vi "To File.vi"(8 "error in":errorcluster, 10 "Filepath":path, 11 "config-ini in":refnum<class "config-ini.lvclass">) -> (0 "error out":errorcluster, 3 "config-ini out":refnum<class "config-ini.lvclass">)   [LabVIEW 2022 SP3, in "hse-config.lvlib" / "config-ini.lvclass"]
doc: "Writes the config-ini object to an INI-file.\n\n____\nHAMPEL SOFTWARE ENGINEERING v3.8.0 (2023-12-18 14:41)"
uses:
  config-ini.lvclass
  <vilib>/Utility/config.llb/Write Key (Boolean).vi
  <vilib>/Utility/config.llb/Write Key (String).vi
  <vilib>/Utility/config.llb/Write Key (Double).vi
  <vilib>/Utility/config.llb/Write Key (I32).vi
  <vilib>/Utility/config.llb/NI_LVConfig.lvlib
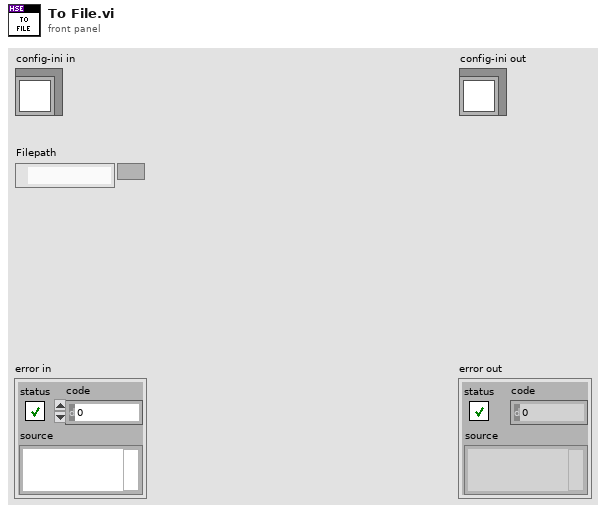
[diagram p1: front panel]
types:
  T1 = typedef "NI_LVConfig.lvlib/Config Data RefNum.ctl" = refnum<k1>
  T2 = typedef "NI_Data Type.lvlib/Data Type.ctl" = enum8{"Invalid Type", "Void", "I8", "I16", "I32", "I64", "U8", "U16", "U32", "U64", "Single Float", "Double Float", "Extended Float", "Single Complex", "Double Complex", "Extended Complex", "Enum U8", "Enum U16", "Enum U32", "Enum U64", "Single Float With Unit", "Double Float With Unit", "Extended Float With Unit", "Single Complex with Unit", "Double Complex with Unit", "Extended Complex with Unit", "Boolean", "String", "Path", "Picture", "Tag", "Array", "Cluster", "Variant", "LV Variant", "Waveform", "Timestamp", "Digital Waveform", "Digital Data", "ExpressData", "Refnum", "External Data", "VI", "Poly VI", "LabVIEW Class Instance", "Fixed Point", "Set Collection", "Map Collection"}
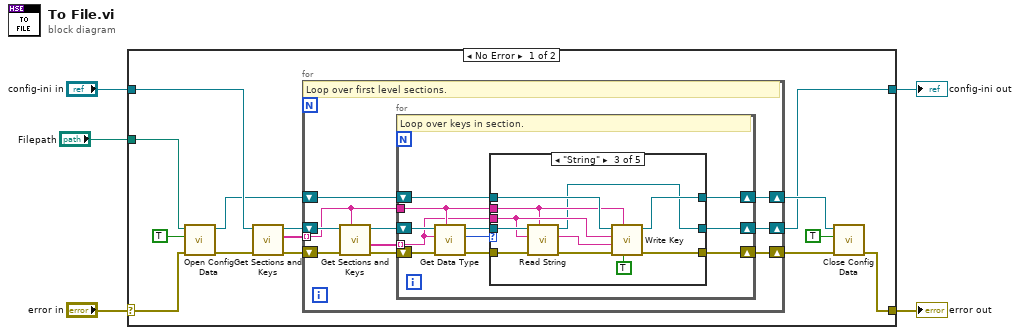
[diagram p0: block diagram]
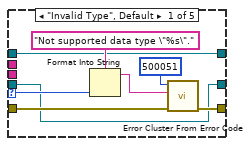
[diagram p2: hidden frame]
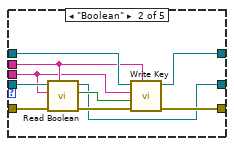
[diagram p3: hidden frame]
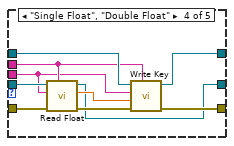
[diagram p4: hidden frame]
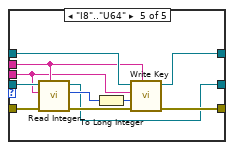
[diagram p5: hidden frame]
diagram:
  n1 = case shown="No Error" "error in" {
    selector: "error in" -> [w19 w92]
    tunnel: [w7 w92] -> w4
    tunnel: [w8 w91] -> w2
    tunnel: "config-ini in" -> [w15 w91]
    tunnel: "Filepath" -> [w18 _]
    frame No Error {
      n2 = call <vilib>:"Open Config Data.vi"("error in (no error)"=w19, "create file if necessary (T)"=TRUE, "configuration file path"=w18) -> ("error out"=w16:errorcluster, "refnum"=w11:T1)  [unwired: 6 in, 1 out]
      n3 = call-dynamic "Get Sections and Keys.vi"("error in"=w16, "config-base in"=w15) -> ("error out"=w14:errorcluster, "Sections"=w13:string[], "config-base out"=w12:refnum<class "config-ini.lvclass">)  [unwired: 5 in, 2 out]
      n4 = for {
        tunnel: w13 -> [w24] mode=indexing
        shift-right: [w22] -> w9
        shift-left: w11 -> [w25]
        shift-right: [w21] -> w8
        shift-left: w12 -> [w28]
        shift-right: [w20] -> w10
        shift-left: w14 -> [w29]
        # "Loop over first level sections."
        n5 = call-dynamic "Get Sections and Keys.vi"("Section"=w24, "error in"=w29, "config-base in"=w28) -> ("error out"=w26:errorcluster, "Keys"=w27:string[], "config-base out"=w23:refnum<class "config-ini.lvclass">)  [unwired: 4 in, 2 out]
        n6 = for {
          tunnel: w27 -> [w33] mode=indexing
          tunnel: w24 -> [w38]
          shift-right: [w31] -> w22
          shift-left: w25 -> [w40]
          shift-right: [w30] -> w21
          shift-left: w23 -> [w39]
          shift-right: [w32] -> w20
          shift-left: w26 -> [w37]
          # "Loop over keys in section."
          n7 = call-dynamic "Get Data Type.vi"("Section"=w38, "error in (no error)"=w37, "Key"=w33, "config-base in"=w39) -> ("error out"=w36:errorcluster, "Data Type"=w35:T2, "config-base out"=w34:refnum<class "config-ini.lvclass">)  [unwired: 5 in]
          n8 = case shown="\"String\"" w35 {
            selector: w35 -> [w44 _ _ _ _]
            tunnel: w40 -> [w42 w58 w69 w79 w90]
            tunnel: w38 -> [_ w52 w63 w73 w82]
            tunnel: w36 -> [w48 w56 w67 w77 w88]
            tunnel: w34 -> [w41 w57 w65 w74 w86]
            tunnel: w33 -> [_ w51 w64 w72 w81]
            tunnel: [w43 w53 w68 w78 w89] -> w32
            tunnel: [w42 w50 w61 w71 w83] -> w31
            tunnel: [w41 w49 w60 w70 w80] -> w30
            frame "Invalid Type", Default {
              n9 = Format Into String(format string="Not supported data type \"%s\"." ("error message (\"\")"), w44) -> (resulting string=w46:string)  [unwired: 2 in, 1 out]
              n10 = call <vilib>:"Error Cluster From Error Code.vi"("error in (no error)"=w48, "error message (\"\")"=w46, "error code (0)"=500051) -> ("error out"=w43:errorcluster)  [unwired: 6 in]
            }
            frame "Boolean" {
              n11 = call-dynamic "Read Boolean.vi"("Section"=w52, "error in"=w56, "Key"=w51, "config-base in"=w57) -> ("error out"=w54:errorcluster, "Value"=w55:bool, "config-base out"=w49:refnum<class "config-ini.lvclass">)  [unwired: 5 in]
              n12 = call-poly <vilib>:"Write Key.vi"("section"=w52, "error in (no error)"=w54, "value"=w55, "key"=w51, "refnum"=w58) -> ("error out"=w53:errorcluster, "refnum out"=w50:T1)  [unwired: 4 in, 1 out]
            }
            frame "String" {
              n13 = call-dynamic "Read String.vi"("Section"=w63, "error in"=w67, "Key"=w64, "config-base in"=w65) -> ("error out"=w66:errorcluster, "Value"=w62:string, "config-base out"=w60:refnum<class "config-ini.lvclass">)  [unwired: 5 in]
              n14 = call-poly <vilib>:"Write Key.vi"("write raw string? (F)"=TRUE, "section"=w63, "error in (no error)"=w66, "value"=w62, "key"=w64, "refnum"=w69) -> ("error out"=w68:errorcluster, "refnum out"=w61:T1)  [unwired: 3 in, 1 out]
            }
            frame "Single Float", "Double Float" {
              n15 = call-dynamic "Read Float.vi"("Section"=w73, "error in"=w77, "Key"=w72, "config-base in"=w74) -> ("error out"=w76:errorcluster, "Value"=w75:dbl, "config-base out"=w70:refnum<class "config-ini.lvclass">)  [unwired: 5 in]
              n16 = call-poly <vilib>:"Write Key.vi"("section"=w73, "error in (no error)"=w76, "value"=w75, "key"=w72, "refnum"=w79) -> ("error out"=w78:errorcluster, "refnum out"=w71:T1)  [unwired: 4 in, 1 out]
            }
            frame "I8".."U64" {
              n17 = call-dynamic "Read Integer.vi"("Section"=w82, "error in"=w88, "Key"=w81, "config-base in"=w86) -> ("error out"=w87:errorcluster, "Value"=w85:i64, "config-base out"=w80:refnum<class "config-ini.lvclass">)  [unwired: 5 in]
              n18 = To Long Integer(number=w85) -> (32bit integer=w84:i32)
              n19 = call-poly <vilib>:"Write Key.vi"("section"=w82, "error in (no error)"=w87, "value"=w84, "key"=w81, "refnum"=w90) -> ("error out"=w89:errorcluster, "refnum out"=w83:T1)  [unwired: 4 in, 1 out]
            }
          }
        }
      }
      n20 = call <vilib>:"Close Config Data.vi"("error in (no error)"=w10, "write file if changed (T)"=TRUE, "refnum"=w9) -> ("error out"=w7:errorcluster)  [unwired: 7 in, 1 out]
    }
    frame Error {
    }
  }
  "error out" <- w4
  "config-ini out" <- w2
